vi "Read (Single Point).vi"(8 "error in (no error)":errorcluster, 11 "VISA resource name":refnum<visa-resource-name>) -> (0 "error out":errorcluster, 2 "Measurement":dbl, 3 "VISA resource name out":refnum<visa-resource-name>)   [LabVIEW 2020, in "PICOTEST M351XA Series.lvlib"]
doc: "Reads and returns single measurement from the instrument. Check the current function of instrument and the measurement, compare the measurement with the function condition and using the fit value and status message before output the measurement."
uses:
  PICOTEST M351XA Series.lvlib
panel:
  in  "General Settings:Timeout Value":u32
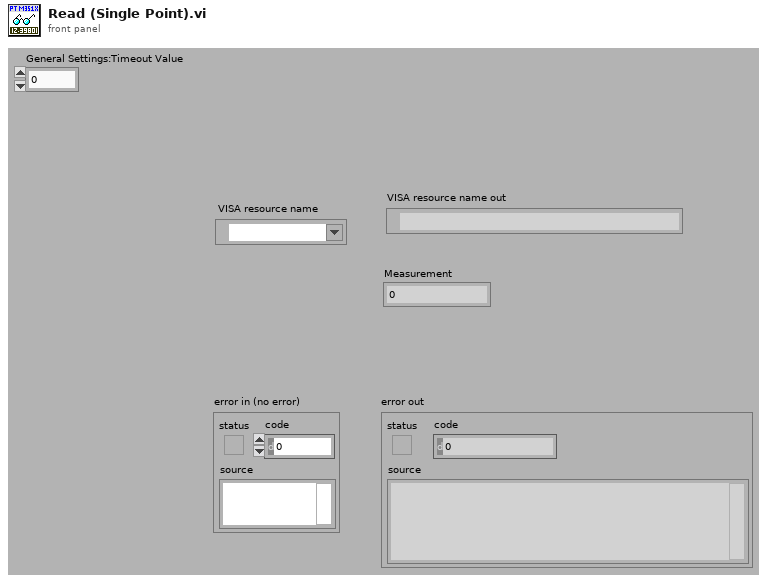
[diagram p1: front panel]
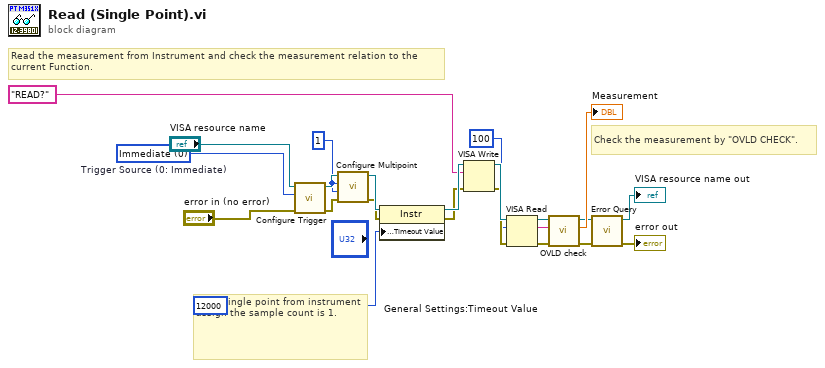
[diagram p0: block diagram]
diagram:
  w9 = u16 0 items=["Immediate", "Software (Bus)", "External"]  # Trigger Source (0: Immediate)
  w10 = 1 ("Sample Count (1)")
  # "Check the measurement by \"OVLD CHECK\"."
  # "Read single point from instrument \nassign the sample count is 1."
  # "Read the measurement from Instrument and check the measurement relation to the current Function."
  n1 = call "Configure Trigger.vi"("error in (no error)"="error in (no error)", "Trigger Source (0: Immediate)"=w9, "VISA resource name"="VISA resource name") -> ("error out"=w12:errorcluster, "VISA resource name out"=w11:refnum<visa-resource-name>)  [unwired: 7 in]
  n2 = call "Configure Multipoint.vi"("error in (no error)"=w12, "Sample Count (1)"=w10, "Trigger Count (1)"=w10, "VISA resource name"=w11) -> ("error out"=w6:errorcluster, "VISA resource name out"=w7:refnum<visa-resource-name>)  [unwired: 6 in]
  n3 = property class="Instr"(reference=w7, error in=w6, "General Settings:Timeout Value"=u32 12000) -> (reference out=w19:refnum<visa-resource-name>, error out=w18:errorcluster)
  n4 = VISA Write(VISA resource name=w19, write buffer="READ?", error in (no error)=w18) -> (VISA resource name out=w23:refnum<visa-resource-name>, error out=w22:errorcluster)  [unwired: 1 out]
  n5 = VISA Read(VISA resource name=w23, byte count=100, error in (no error)=w22) -> (VISA resource name out=w17:refnum<visa-resource-name>, read buffer=w15:string, error out=w16:errorcluster)  [unwired: 1 out]
  n6 = call "OVLD check.vi"("error in (no error)"=w16, "Measurement (in)"=w15, "VISA resource name"=w17) -> ("error out"=w2:errorcluster, "Measurement (out)"=→"Measurement":dbl, "VISA resource name out"=w1:refnum<visa-resource-name>)  [unwired: 6 in]
  n7 = call "Error Query.vi"("error in (no error)"=w2, "VISA resource name"=w1) -> ("error out"=→"error out":errorcluster, "VISA resource name out"=→"VISA resource name out":refnum<visa-resource-name>)  [unwired: 6 in, 2 out]
